vi "String to Scrolling Message Array.vi"(10 "LCD Displayable Characters Number":u8=16, 11 "String To Display:":string="Made using LabVIEW") -> (2 "Scrollable Messages Array Size":i32, 3 "Scrolling Messages Array":string[](array[string]))   [LabVIEW 2021]
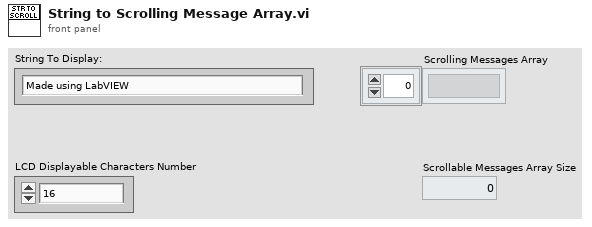
[diagram p1: front panel]
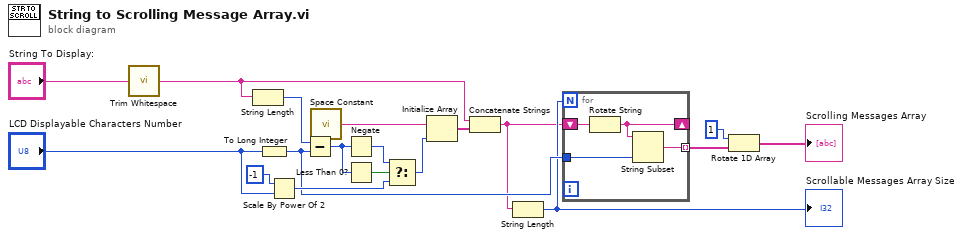
[diagram p0: block diagram]
diagram:
  n1 = call <vilib>:"Trim Whitespace.vi"("string"="String To Display:") -> ("trimmed string"=w4:string)  [unwired: 1 in]
  n2 = String Length(string=w4) -> (length=w5:i32)
  n3 = To Long Integer(number="LCD Displayable Characters Number") -> (32bit integer=w15:i32)
  n4 = Scale By Power Of 2(n=i16 -1, x="LCD Displayable Characters Number") -> (x*2^n=w18:u8)
  n5 = Subtract(x=w5, y=w15) -> (x-y=w6:i32)
  n6 = call <vilib>:"Space Constant.vi"() -> ("String"=w2:string)
  n7 = Negate(x=w6) -> (-x=w7:i32)
  n8 = Less Than 0?(x=w6) -> (x < 0?=w9:bool)
  n9 = Select(t=w7, s=w9, f=w18) -> (s? t:f=w8:i32)
  n10 = Initialize Array(w2, w8) -> (w3:string[])
  n11 = Concatenate Strings(w4, w3) -> (w10:string)
  n12 = String Length(string=w10) -> (length=w14:i32)
  "Scrollable Messages Array Size" <- w14
  n13 = for {
    N: w14 -> [_]
    shift-right: [w21] -> _
    shift-left: w10 -> [w22]
    tunnel: [w20] -> w11 mode=indexing
    tunnel: w15 -> [w19]
    n14 = Rotate String(1:w22) -> (0:w21:string)
    n15 = String Subset(string=w21, length (rest)=w19) -> (substring=w20:string)  [unwired: 1 in]
  }
  n16 = Rotate 1D Array(1:w11, 2:1 ("n")) -> (0:→"Scrolling Messages Array":string[])
